vi "Real Pool navigation demo.vi"() -> ()   [LabVIEW 2011]
panel:
  in  "Image file name":string="real pool targets rotated.bmp"
  out "Whale":cluster{"x":sgl, "y":sgl}
  out "Bouy":cluster{"x":sgl, "y":sgl}
  out "Boat":cluster{"x":sgl, "y":sgl}
  out "Boat\nHeading":sgl
  out "Location":cluster{"x":sgl, "y":sgl}
  in  "stop":bool
  out "error out":errorcluster
  out "Working Image":T1(plugin-control)
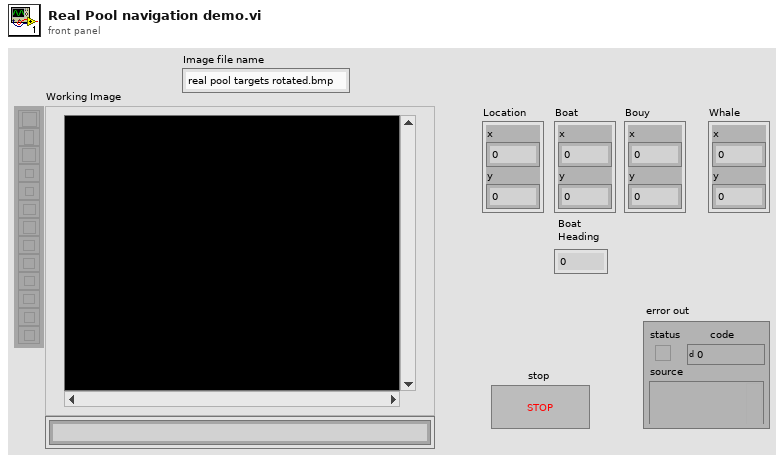
[diagram p1: front panel]
types:
  T1 = typedef "IMAQ Image.ctl" = refnum<image>
  T2 = typedef "Image Type" = u32
  T3 = typedef "IMAQ GM Match Report.ctl" = cluster{"Position":cluster{"x":sgl, "y":sgl}, "Angle":sgl, "Scale":sgl, "Score":sgl, "Bounding Box":cluster{"x":sgl, "y":sgl}[], "Contrast Reversed":bool, "Occlusion %":sgl, "Template Target Curve Score":sgl, "Target Template Curve Score":sgl, "Correlation Score":sgl}
  T4 = cluster{"Position":cluster{"x":sgl, "y":sgl}, "Angle":sgl, "Scale":sgl, "Score":sgl, "Bounding Box":cluster{"x":sgl, "y":sgl}[]}[]
  T5 = cluster{"Position":cluster{"x":sgl, "y":sgl}, "Angle":sgl, "Scale":sgl, "Score":sgl, "Bounding Box":cluster{"x":sgl, "y":sgl}[]}
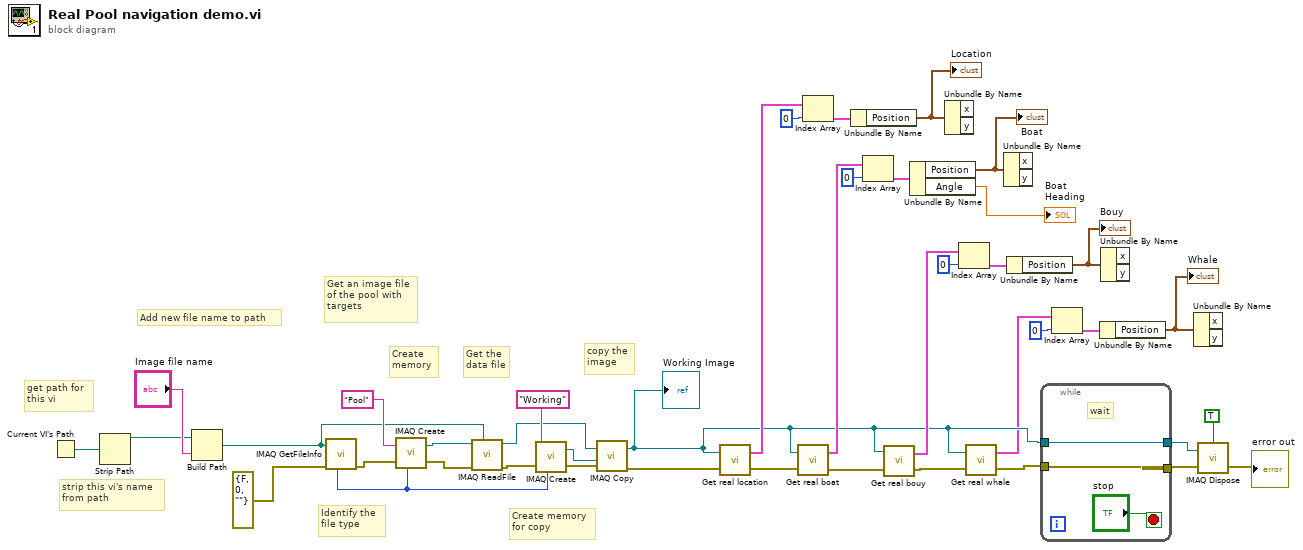
[diagram p0: block diagram]
diagram:
  # "Create memory\nfor copy"
  # "copy the\nimage"
  # "Add new file name to path"
  # "strip this vi's name \nfrom path"
  # "get path for \nthis vi"
  # "Get the \ndata file"
  # "Create \nmemory"
  # "Identify the \nfile type"
  # "Get an image file\nof the pool with\ntargets"
  n1 = Current VI's Path() -> (path=w33:path)
  n2 = Strip Path(path=w33) -> (stripped path=w32:path)  [unwired: 1 out]
  n3 = Build Path(base path=w32, name or relative path="Image file name") -> (appended path=w31:path)
  n4 = call "IMAQ GetFileInfo"("error in (no error)"=errorcluster {"status"=FALSE, "code"=0, "source"=""}, "File Path"=w31) -> ("error out"=w42:errorcluster, "Image Type"=w4:T2)  [unwired: 3 in, 5 out]
  n5 = call "IMAQ Create"("Image Name"="Pool", "Image Type"=w4, "error in (no error)"=w42) -> ("New Image"=w40:T1, "error out"=w37:errorcluster)  [unwired: 2 in]
  n6 = call "IMAQ ReadFile"("File Path"=w31, "error in (no error)"=w37, "Image"=w40) -> ("error out"=w5:errorcluster, "Image Out"=w26:T1)  [unwired: 4 in, 3 out]
  n7 = call "IMAQ Create"("Image Name"="Working", "Image Type"=w4, "error in (no error)"=w5) -> ("New Image"=w35:T1, "error out"=w38:errorcluster)  [unwired: 2 in]
  n8 = call "IMAQ Copy"("error in (no error)"=w38, "Image Dst"=w35, "Image Src"=w26) -> ("error out"=w3:errorcluster, "Image Dst Out"=w2:T1)  [unwired: 3 in]
  "Working Image" <- w2
  n9 = call "Get real location.vi"("error in"=w3, "Image"=w2) -> ("error out"=w22:errorcluster, "Matches"=w23:T3[])
  n10 = call "Get real boat.vi"("error in"=w22, "Image"=w2) -> ("error out"=w15:errorcluster, "Matches"=w16:T3[])
  n11 = Index Array(array=w23, index=0) -> (element=w25:T3)
  n12 = Unbundle By Name(w25) -> ("Position"=w24:cluster{"x":sgl, "y":sgl})
  "Location" <- w24
  n13 = Index Array(array=w16, index=0) -> (element=w20:T3)
  n14 = call "Get real bouy.vi"("error in"=w15, "Image"=w2) -> ("error out"=w10:errorcluster, "Matches"=w11:T3[])
  n15 = Unbundle By Name(w20) -> ("Position"=w19:cluster{"x":sgl, "y":sgl}, "Angle"=→"Boat\nHeading":sgl)
  "Boat" <- w19
  n16 = Unbundle By Name(w24) -> ()  [unwired: 2 out]
  n17 = Index Array(array=w11, index=0) -> (element=w13:T3)
  n18 = call "Get real whale.vi"("error in"=w10, "Image"=w2) -> ("error out"=w9:errorcluster, "Matches"=w1:T4)
  n19 = Unbundle By Name(w19) -> ()  [unwired: 2 out]
  n20 = Unbundle By Name(w13) -> ("Position"=w12:cluster{"x":sgl, "y":sgl})
  "Bouy" <- w12
  n21 = while {
    tunnel: w2 -> [w43]
    tunnel: w9 -> [w44]
    tunnel: [w44] -> w30
    tunnel: [w43] -> w28
    stop <- "stop" stop-if-true
    # "wait"
  }
  n22 = Index Array(array=w1, index=0) -> (element=w8:T5)
  n23 = Unbundle By Name(w8) -> ("Position"=w7:cluster{"x":sgl, "y":sgl})
  "Whale" <- w7
  n24 = Unbundle By Name(w12) -> ()  [unwired: 2 out]
  n25 = Unbundle By Name(w7) -> ()  [unwired: 2 out]
  n26 = call "IMAQ Dispose"("All Images? (No)"=TRUE, "Image"=w28, "error in (no error)"=w30) -> ("error out"=→"error out":errorcluster)  [unwired: 3 in]
